vi "Autonomous Independent.vi"() -> ()   [LabVIEW 2015]
doc: "This VI is called when autonomous begins, and will automatically be terminated when autonomous ends. You can carry out timed or sensor driven robot movement independently without needing to return to the caller."
uses:
  <vilib>/Rock Robotics/WPI/SafetyOutput/WPI_SafetyOutputConfigMenu.ctl
  <vilib>/Rock Robotics/Network Tables/NT Read Number.vi
  <vilib>/Rock Robotics/WPI/Utilities/WPI_GetSetVariantRefNum.vi
  <vilib>/Rock Robotics/WPI/Solenoid/Deprecated/WPI_SolenoidGetBool.vi
  <vilib>/Rock Robotics/WPI/Solenoid/Deprecated/WPI_SolenoidSetBool.vi
panel:
  in  "Far":dbl=0.7
  in  "Close":dbl=0.7
  in  "Right Offset":dbl=1.0
  out "Defense Type":dbl=3.0
  in  "Auton_Modes":T1(array[cluster])=[{"Actions"=[{"Action"=enum."Drive", "Effort"=0.55, "Duration"=3.5}, {"Action"=enum."Nothing", "Effort"=0.0, "Duration"=0.0}]}, {"Actions"=[{"Action"=enum."Art Down", "Effort"=0.0, "Duration"=1.0}, {"Action"=enum."Drive", "Effort"=0.75, "Duration"=5.0}, {"Action"=enum."Art Up", "Effort"=0.0, "Duration"=1.0}]}, {"Actions"=[{"Action"=enum."Drive", "Effort"=1.0, "Duration"=3.0}, {"Action"=enum."Art Down", "Effort"=0.0, "Duration"=1.0}, {"Action"=enum."Drive", "Effort"=0.75, "Duration"=3.5}, {"Action"=enum."Art Up", "Effort"=0.0, "Duration"=1.0}]}, {"Actions"=[{"Action"=enum."Art Down", "Effort"=0.0, "Duration"=0.5}, {"Action"=enum."Drive", "Effort"=0.8, "Duration"=5.28}, {"Action"=enum."Art Up", "Effort"=0.0, "Duration"=1.0}, {"Action"=enum."Turn", "Effort"=-0.8, "Duration"=1.8}, {"Action"=enum."Nothing", "Effort"=0.0, "Duration"=0.1}, {"Action"=enum."Drive", "Effort"=0.8, "Duration"=1.75}, {"Action"=enum."Art Down", "Effort"=0.0, "Duration"=0.5}, {"Action"=enum."Vision Shot", "Effort"=0.0, "Duration"=4.0}]}, {"Actions"=[{"Action"=enum."Shift", "Effort"=0.0, "Duration"=0.0}, {"Action"=enum."Drive", "Effort"=1.0, "Duration"=0.1}, {"Action"=enum."Nothing", "Effort"=0.0, "Duration"=0.1}, {"Action"=enum."Drive", "Effort"=1.0, "Duration"=3.0}]}, {"Actions"=[{"Action"=enum."Shift", "Effort"=0.0, "Duration"=0.0}, {"Action"=enum."Drive", "Effort"=1.0, "Duration"=0.1}, {"Action"=enum."Nothing", "Effort"=0.0, "Duration"=0.1}, {"Action"=enum."Drive", "Effort"=1.0, "Duration"=3.0}]}, {"Actions"=[{"Action"=enum."Drive", "Effort"=0.55, "Duration"=4.0}, {"Action"=enum."Art Down", "Effort"=0.0, "Duration"=1.0}, {"Action"=enum."Drive", "Effort"=-0.5, "Duration"=0.6}, {"Action"=enum."Drive", "Effort"=0.75, "Duration"=1.0}, {"Action"=enum."Art Up", "Effort"=0.0, "Duration"=1.0}, {"Action"=enum."Drive", "Effort"=0.75, "Duration"=3.0}]}, {"Actions"=[{"Action"=enum."Art Down", "Effort"=0.0, "Duration"=0.5}, {"Action"=enum."Drive", "Effort"=0.55, "Duration"=4.25}, {"Action"=enum."Art Up", "Effort"=0.0, "Duration"=0.0}, {"Action"=enum."Nothing", "Effort"=0.0, "Duration"=0.3}, {"Action"=enum."Drive", "Effort"=0.9, "Duration"=2.0}]}, {"Actions"=[{"Action"=enum."Nothing", "Effort"=0.0, "Duration"=0.0}]}]
  # "0 Reach Defense\n1 Low Bar\n2 Rough Terrain\n3 Moat\n4 Rock Wall\n5 Ramparts\n6 Cheval\n7 Portcullis\n8 None"
  # "Reach"
  # "Low Bar"
  # "Rough Terrain"
  # "Moat"
  # "Low Bar \nVision"
  # "Rockwall"
  # "Left Side \nCheval w/\nTarget"
  # "Ramparts"
  # "Right Side \nCheval w/\ntarget"
  # "Cheval"
  # "Portcullis"
  # "None"
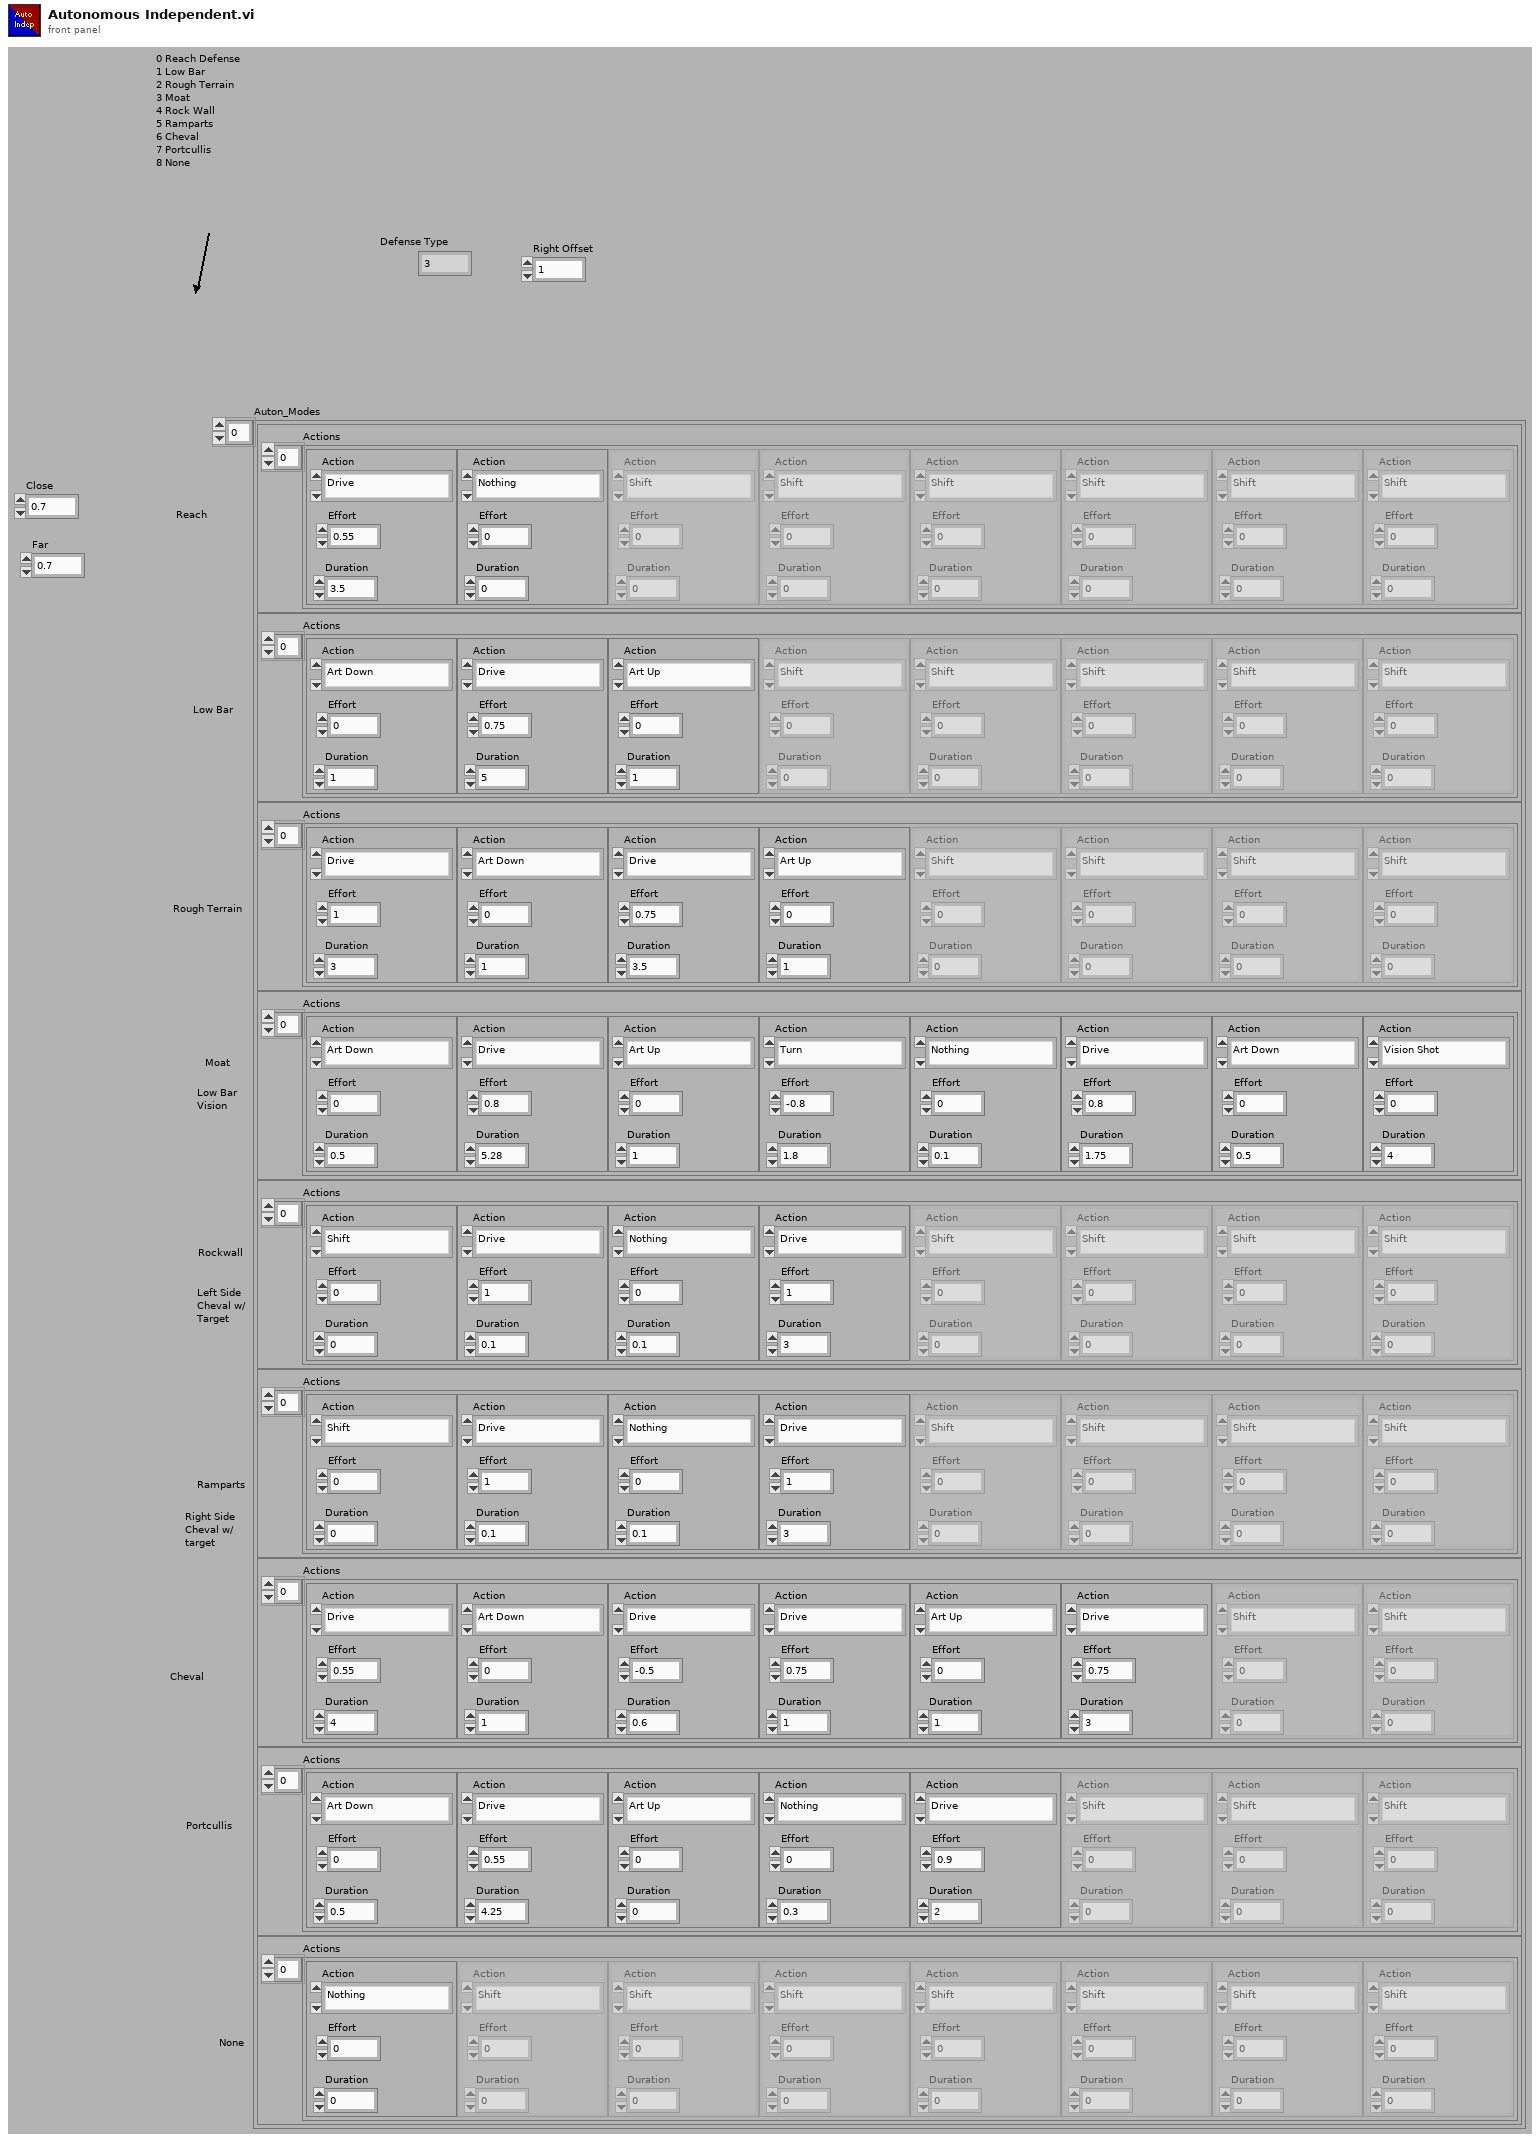
[diagram p1: front panel]
types:
  T1 = cluster{"Actions":cluster{"Action":enum16{"Shift", "Shoot", "Move Articulates", "Nothing", "Drive", "Turn", "Vision Shot", "Art Up", "Art Down", "Test"}, "Effort":dbl, "Duration":dbl}[]}[]
  T2 = cluster{"Actions":cluster{"Action":enum16{"Shift", "Shoot", "Move Articulates", "Nothing", "Drive", "Turn", "Vision Shot", "Art Up", "Art Down", "Test"}, "Effort":dbl, "Duration":dbl}[]}
  T3 = cluster{"Action":enum16{"Shift", "Shoot", "Move Articulates", "Nothing", "Drive", "Turn", "Vision Shot", "Art Up", "Art Down", "Test"}, "Effort":dbl, "Duration":dbl}[]
  T4 = typedef "WPI_SafetyOutputConfigMenu.ctl" = enum16{"Enable", "Disable"}
  T5 = enum16{"Shift", "Shoot", "Move Articulates", "Nothing", "Drive", "Turn", "Vision Shot", "Art Up", "Art Down", "Test"}
  T6 = typedef "WPI_RobotDriveDevRef.ctl" = cluster{"DevStatus":errorcluster, "Motors[]":T7[], "Square Inputs":bool, "Max Output":dbl}
  T7 = typedef "WPI_MotorControlDeviceRef.ctl" = cluster{"DeviceStatus":errorcluster, "Type":T8, "PWM":cluster{"PWM Channel":T9, "DeadBand":T10}, "CAN":cluster{"Device Number":u8, "Control Mode":T11, "Semaphore":T12, "Max Vout":dbl, "TalonSRX Control Mode":T13}, "Invert":bool}
  T8 = typedef "WPI_MotorControlType.ctl" = enum16{"PWM", "CAN", "CANTalonSRX"}
  T9 = typedef "FPGA_DIOPWMChannel.ctl" = enum8{"PWM 0", "PWM 1", "PWM 2", "PWM 3", "PWM 4", "PWM 5", "PWM 6", "PWM 7", "PWM 8", "PWM 9", "PWM MXP 0", "PWM MXP 1", "PWM MXP 2", "PWM MXP 3", "PWM MXP 4", "PWM MXP 5", "PWM MXP 6", "PWM MXP 7", "PWM MXP 8", "PWM MXP 9", "Invalid"}
  T10 = typedef "WPI_PWMDeadband.ctl" = cluster{"Name":string, "maxPositivePwm":i32, "minPositivePwm":i32, "centerPwm":i32, "maxNegativePwm":i32, "minNegativePwm":i32, "angularRange":u16}
  T11 = typedef "WPI_CANJaguar_ControlMode.ctl" = enum8{"Percent VBus", "Current", "Speed", "Position", "Voltage"}
  T12 = typedef "Semaphore RefNum" = refnum<k1>
  T13 = typedef "WPI_CANTalonSRX_APIControlMode.ctl" = enum8{"Percent VBus", "Speed", "Position", "Slave", "Unchanged / Invalid", "Voltage Compensation", "Current", "Motion Profile"}
  T14 = typedef "WPI_SolenoidDevRef.ctl" = cluster{"DevStatus":errorcluster, "Pneumatics Control Module":u8, "Forward Solenoid Channel":T15, "Reverse Solenoid Channel":T15}
  T15 = typedef "WPI_SolenoidChannel.ctl" = enum8{"Solenoid 0", "Solenoid 1", "Solenoid 2", "Solenoid 3", "Solenoid 4", "Solenoid 5", "Solenoid 6", "Solenoid 7", "Invalid"}
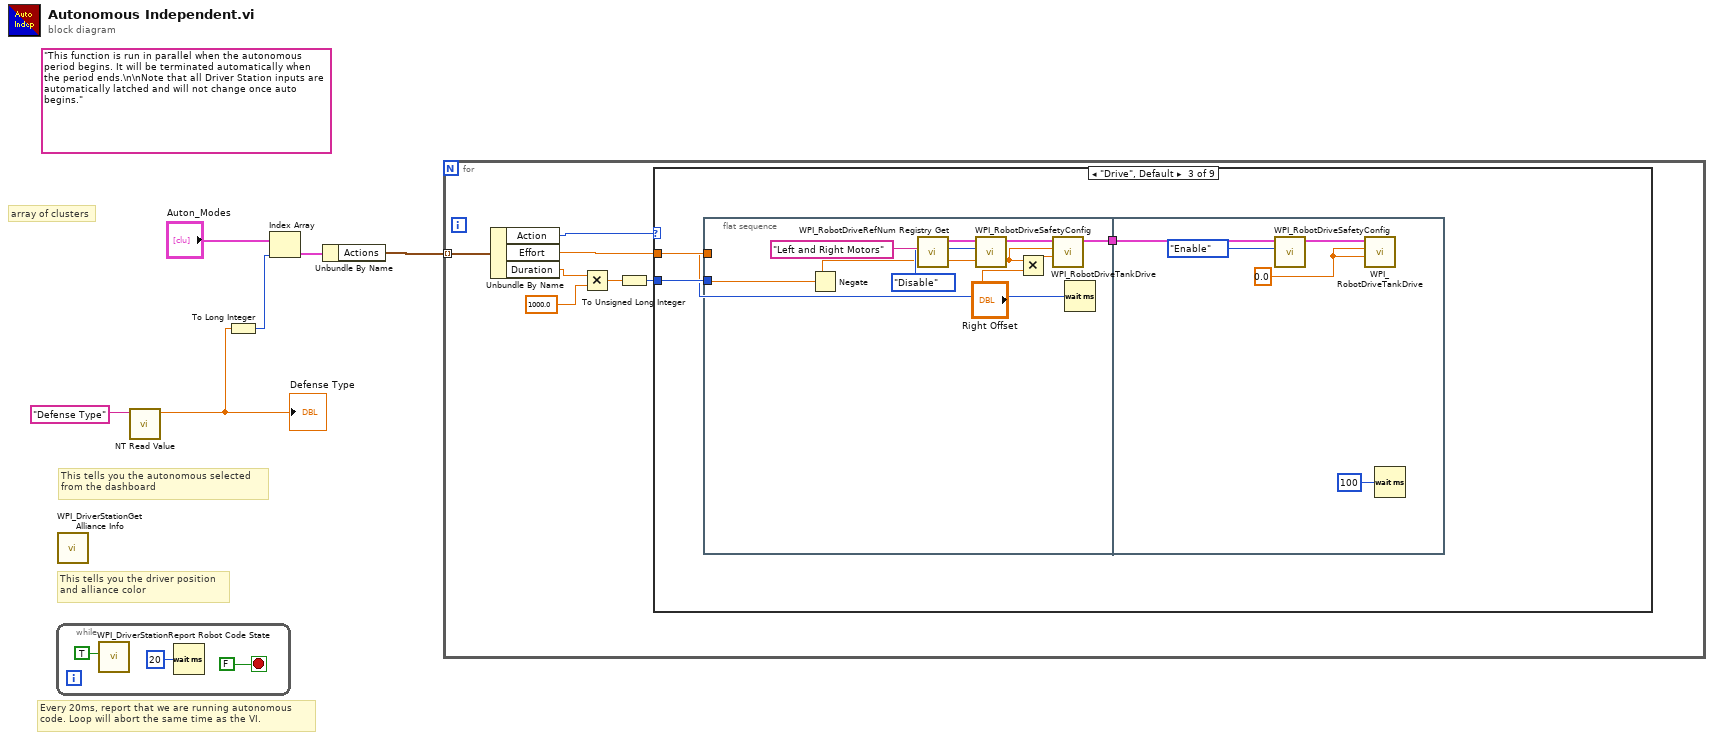
[diagram p0: block diagram]
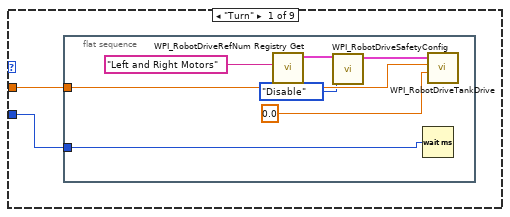
[diagram p2: hidden frame]
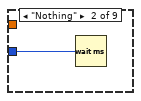
[diagram p3: hidden frame]
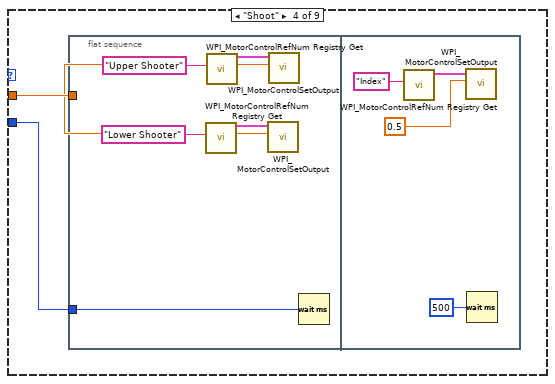
[diagram p4: hidden frame]
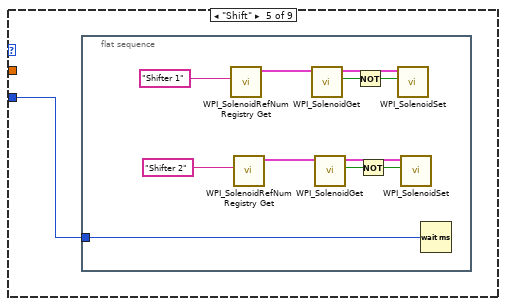
[diagram p5: hidden frame]
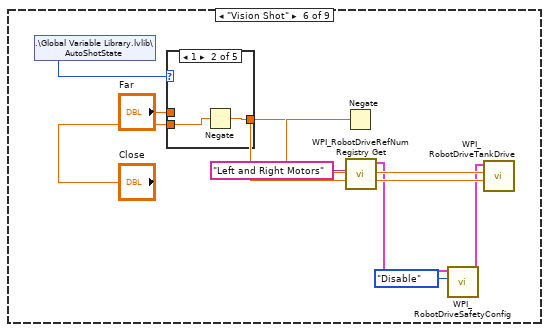
[diagram p6: hidden frame]
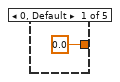
[diagram p7: hidden frame]
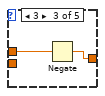
[diagram p8: hidden frame]
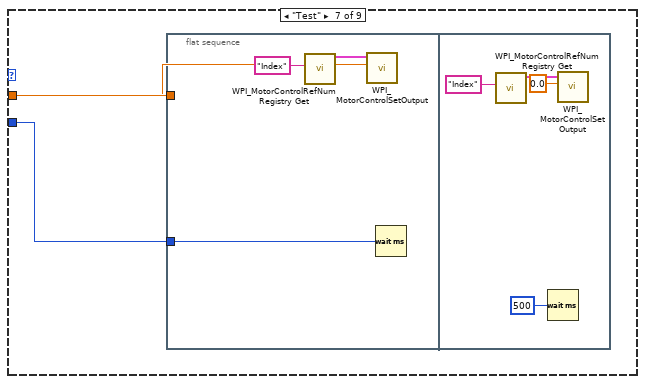
[diagram p11: hidden frame]
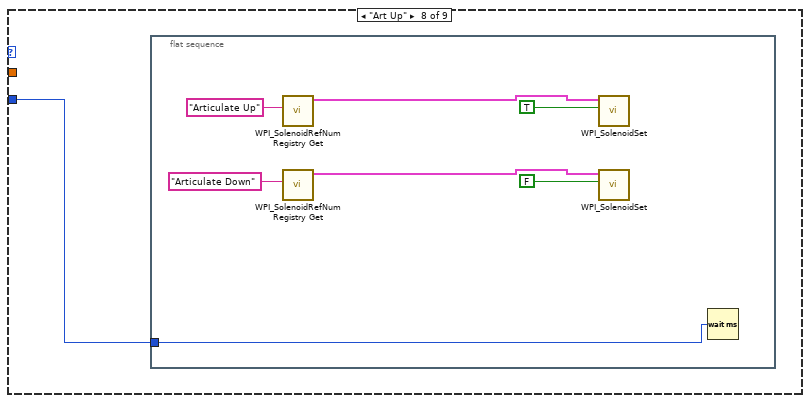
[diagram p12: hidden frame]
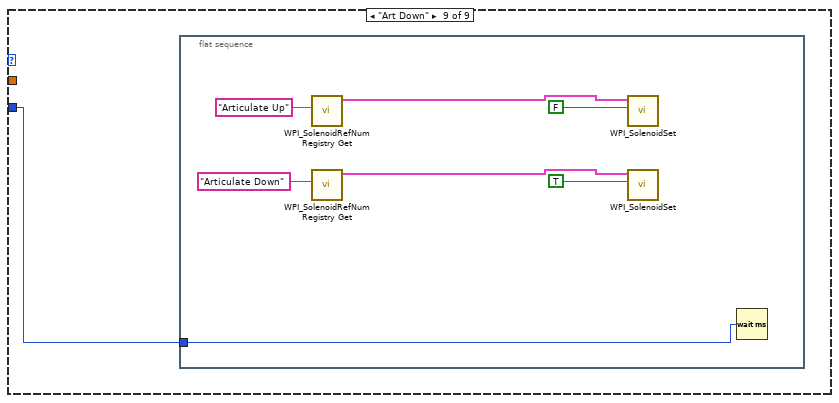
[diagram p13: hidden frame]
diagram:
  (unwired) "This function is run in parallel when the autonomous period begins. It will be terminated automatically when the period ends.\n\nNote that all Driver Station inputs are automatically latched and will not change once auto begins."
  # "This tells you the autonomous selected\nfrom the dashboard"
  # "array of clusters"
  # "Every 20ms, report that we are running autonomous\ncode. Loop will abort the same time as the VI."
  # "This tells you the driver position\nand alliance color"
  n1 = while {
    stop <- FALSE stop-if-true
    n2 = call <vilib>:"WPI_DriverStationReport Robot Code State.vi"("Autonomous"=TRUE) -> ()  [unwired: 10 in, 1 out]
    n3 = Wait (ms)(milliseconds to wait=u32 20) -> ()  [unwired: 1 out]
  }
  n4 = call <vilib>:"WPI_DriverStationGet Alliance Info.vi"() -> ()  [unwired: 12 out]
  n5 = call-poly <vilib>:"NT Read Value.vi"("Name"="Defense Type") -> ("Numeric"=w1:dbl)  [unwired: 9 in, 1 out]
  "Defense Type" <- w1
  n6 = To Long Integer(number=w1) -> (32bit integer=w3:i32)
  n7 = Index Array(array="Auton_Modes", index=w3) -> (element=w5:T2)
  n8 = Unbundle By Name(w5) -> ("Actions"=w6:T3)
  n9 = for {
    tunnel: w6 -> [w16] mode=indexing
    n10 = Unbundle By Name(w16) -> ("Action"=w15:T5, "Effort"=w14:dbl, "Duration"=w13:dbl)
    n11 = Multiply(x=w13, y=1000.0) -> (x*y=w10:dbl)
    n12 = To Unsigned Long Integer(number=w10) -> (unsigned 32bit integer=w11:u32)
    n13 = case shown="\"Drive\", Default" w15 {
      tunnel: w14 -> [w18 _ w29 w45 _ _ w86 _ _]
      tunnel: w11 -> [w17 w26 w28 w46 w57 _ w85 w95 w103]
      frame "Turn" {
        n14 = flat-sequence {
          tunnel: w18 -> [w23]
          tunnel: w17 -> [w24]
          frame #0 {
            n15 = call <vilib>:"WPI_RobotDriveRefNum Registry Get.vi"("refnum name"="Left and Right Motors") -> ("RobotDriveDevRef"=w21:T6)  [unwired: 9 in, 1 out]
            n16 = call <vilib>:"WPI_RobotDriveSafetyConfig.vi"("mode"=WPI_SafetyOutputConfigMenu."Disable", "RobotDriveDevRef"=w21) -> ("RobotDriveDevRef"=w20:T6)  [unwired: 8 in, 1 out]
            n17 = Wait (ms)(milliseconds to wait=w24) -> ()  [unwired: 1 out]
            n18 = call <vilib>:"WPI_RobotDriveTankDrive.vi"("Right axis value"=0.0, "Left axis value"=w23, "RobotDriveDevRef"=w20) -> ()  [unwired: 6 in, 3 out]
          }
        }
      }
      frame "Nothing" {
        n19 = Wait (ms)(milliseconds to wait=w26) -> ()  [unwired: 1 out]
      }
      frame "Drive", Default {
        n20 = flat-sequence {
          tunnel: w29 -> [w37]
          tunnel: w28 -> [w36]
          tunnel: [w35] -> w27
          tunnel: w27 -> [w42]
          frame #0 {
            n21 = Negate(x=w37) -> (-x=w31:dbl)
            n22 = call <vilib>:"WPI_RobotDriveRefNum Registry Get.vi"("refnum name"="Left and Right Motors") -> ("RobotDriveDevRef"=w38:T6)  [unwired: 9 in, 1 out]
            n23 = call <vilib>:"WPI_RobotDriveSafetyConfig.vi"("mode"=WPI_SafetyOutputConfigMenu."Disable", "RobotDriveDevRef"=w38) -> ("RobotDriveDevRef"=w34:T6)  [unwired: 8 in, 1 out]
            n24 = Multiply(x=w31, y="Right Offset") -> (x*y=w32:dbl)
            n25 = call <vilib>:"WPI_RobotDriveTankDrive.vi"("Right axis value"=w32, "Left axis value"=w31, "RobotDriveDevRef"=w34) -> ("RobotDriveDevRef"=w35:T6)  [unwired: 6 in, 2 out]
            n26 = Wait (ms)(milliseconds to wait=w36) -> ()  [unwired: 1 out]
          }
          frame #1 {
            w44 = 0.0
            n27 = call <vilib>:"WPI_RobotDriveSafetyConfig.vi"("mode"=WPI_SafetyOutputConfigMenu."Enable", "RobotDriveDevRef"=w42) -> ("RobotDriveDevRef"=w41:T6)  [unwired: 8 in, 1 out]
            n28 = call <vilib>:"WPI_RobotDriveTankDrive.vi"("Right axis value"=w44, "Left axis value"=w44, "RobotDriveDevRef"=w41) -> ()  [unwired: 6 in, 3 out]
            n29 = Wait (ms)(milliseconds to wait=u32 100) -> ()  [unwired: 1 out]
          }
        }
      }
      frame "Shoot" {
        n30 = flat-sequence {
          tunnel: w46 -> [w47]
          tunnel: w45 -> [w48]
          frame #0 {
            n31 = call <vilib>:"WPI_MotorControlRefNum Registry Get.vi"("refnum name"="Lower Shooter") -> ("MotorControlDevRef"=w49:T7)  [unwired: 9 in, 1 out]
            n32 = call <vilib>:"WPI_MotorControlRefNum Registry Get.vi"("refnum name"="Upper Shooter") -> ("MotorControlDevRef"=w52:T7)  [unwired: 9 in, 1 out]
            n33 = call <vilib>:"WPI_MotorControlSetOutput.vi"("Output"=w48, "MotorControlDevRef"=w49) -> ()  [unwired: 7 in, 3 out]
            n34 = call <vilib>:"WPI_MotorControlSetOutput.vi"("Output"=w48, "MotorControlDevRef"=w52) -> ()  [unwired: 7 in, 3 out]
            n35 = Wait (ms)(milliseconds to wait=w47) -> ()  [unwired: 1 out]
          }
          frame #1 {
            n36 = call <vilib>:"WPI_MotorControlRefNum Registry Get.vi"("refnum name"="Index") -> ("MotorControlDevRef"=w55:T7)  [unwired: 9 in, 1 out]
            n37 = call <vilib>:"WPI_MotorControlSetOutput.vi"("Output"=0.5, "MotorControlDevRef"=w55) -> ()  [unwired: 7 in, 3 out]
            n38 = Wait (ms)(milliseconds to wait=u32 500) -> ()  [unwired: 1 out]
          }
        }
      }
      frame "Shift" {
        n39 = flat-sequence {
          tunnel: w57 -> [w58]
          frame #0 {
            n40 = call <vilib>:"WPI_SolenoidRefNum Registry Get.vi"("refnum name"="Shifter 1") -> ("SolenoidDevRef"=w68:T14)  [unwired: 9 in, 1 out]
            n41 = call <vilib>:"WPI_SolenoidRefNum Registry Get.vi"("refnum name"="Shifter 2") -> ("SolenoidDevRef"=w59:T14)  [unwired: 9 in, 1 out]
            n42 = call-poly <vilib>:"WPI_SolenoidGet.vi"("SolenoidDevRef"=w68) -> ("Value"=w66:bool, "SolenoidDevRef"=w67:T14)  [unwired: 8 in, 1 out]
            n43 = call-poly <vilib>:"WPI_SolenoidGet.vi"("SolenoidDevRef"=w59) -> ("Value"=w61:bool, "SolenoidDevRef"=w60:T14)  [unwired: 8 in, 1 out]
            n44 = Not(x=w66) -> (.not. x?=w64:bool)
            n45 = Not(x=w61) -> (.not. x?=w63:bool)
            n46 = call-poly <vilib>:"WPI_SolenoidSet.vi"("Value"=w64, "SolenoidDevRef"=w67) -> ()  [unwired: 8 in, 2 out]
            n47 = call-poly <vilib>:"WPI_SolenoidSet.vi"("Value"=w63, "SolenoidDevRef"=w60) -> ()  [unwired: 8 in, 2 out]
            n48 = Wait (ms)(milliseconds to wait=w58) -> ()  [unwired: 1 out]
          }
        }
      }
      frame "Vision Shot" {
        n49 = shared-variable ".\\Global Variable Library.lvlib\\AutoShotState"() -> (w75:u32)  [unwired: 1 in, 1 out]
        n50 = case shown="1" w75 {
          tunnel: [0.0 w80 w82 w83 w84] -> w72
          tunnel: "Far" -> [_ _ w81 _ w84]
          tunnel: "Close" -> [_ w79 _ w83 _]
          frame 0, Default {
          }
          frame 1 {
            n51 = Negate(x=w79) -> (-x=w80:dbl)
          }
          frame 3 {
            n52 = Negate(x=w81) -> (-x=w82:dbl)
          }
          frame 4 {
          }
          frame 6 {
          }
        }
        n53 = Negate(x=w72) -> (-x=w77:dbl)
        n54 = call <vilib>:"WPI_RobotDriveRefNum Registry Get.vi"("refnum name"="Left and Right Motors") -> ("RobotDriveDevRef"=w71:T6)  [unwired: 9 in, 1 out]
        n55 = call <vilib>:"WPI_RobotDriveSafetyConfig.vi"("mode"=WPI_SafetyOutputConfigMenu."Disable", "RobotDriveDevRef"=w71) -> ("RobotDriveDevRef"=w70:T6)  [unwired: 8 in, 1 out]
        n56 = call <vilib>:"WPI_RobotDriveTankDrive.vi"("Right axis value"=w72, "Left axis value"=w77, "RobotDriveDevRef"=w70) -> ()  [unwired: 6 in, 3 out]
      }
      frame "Test" {
        n57 = flat-sequence {
          tunnel: w86 -> [w88]
          tunnel: w85 -> [w87]
          frame #0 {
            n58 = call <vilib>:"WPI_MotorControlRefNum Registry Get.vi"("refnum name"="Index") -> ("MotorControlDevRef"=w90:T7)  [unwired: 9 in, 1 out]
            n59 = call <vilib>:"WPI_MotorControlSetOutput.vi"("Output"=w88, "MotorControlDevRef"=w90) -> ()  [unwired: 7 in, 3 out]
            n60 = Wait (ms)(milliseconds to wait=w87) -> ()  [unwired: 1 out]
          }
          frame #1 {
            n61 = call <vilib>:"WPI_MotorControlRefNum Registry Get.vi"("refnum name"="Index") -> ("MotorControlDevRef"=w93:T7)  [unwired: 9 in, 1 out]
            n62 = Wait (ms)(milliseconds to wait=u32 500) -> ()  [unwired: 1 out]
            n63 = call <vilib>:"WPI_MotorControlSetOutput.vi"("Output"=0.0, "MotorControlDevRef"=w93) -> ()  [unwired: 7 in, 3 out]
          }
        }
      }
      frame "Art Up" {
        n64 = flat-sequence {
          tunnel: w95 -> [w96]
          frame #0 {
            n65 = call <vilib>:"WPI_SolenoidRefNum Registry Get.vi"("refnum name"="Articulate Up") -> ("SolenoidDevRef"=w100:T14)  [unwired: 9 in, 1 out]
            n66 = call <vilib>:"WPI_SolenoidRefNum Registry Get.vi"("refnum name"="Articulate Down") -> ("SolenoidDevRef"=w97:T14)  [unwired: 9 in, 1 out]
            n67 = call-poly <vilib>:"WPI_SolenoidSet.vi"("Value"=TRUE, "SolenoidDevRef"=w100) -> ()  [unwired: 8 in, 2 out]
            n68 = call-poly <vilib>:"WPI_SolenoidSet.vi"("Value"=FALSE, "SolenoidDevRef"=w97) -> ()  [unwired: 8 in, 2 out]
            n69 = Wait (ms)(milliseconds to wait=w96) -> ()  [unwired: 1 out]
          }
        }
      }
      frame "Art Down" {
        n70 = flat-sequence {
          tunnel: w103 -> [w104]
          frame #0 {
            n71 = call <vilib>:"WPI_SolenoidRefNum Registry Get.vi"("refnum name"="Articulate Up") -> ("SolenoidDevRef"=w108:T14)  [unwired: 9 in, 1 out]
            n72 = call <vilib>:"WPI_SolenoidRefNum Registry Get.vi"("refnum name"="Articulate Down") -> ("SolenoidDevRef"=w105:T14)  [unwired: 9 in, 1 out]
            n73 = call-poly <vilib>:"WPI_SolenoidSet.vi"("Value"=FALSE, "SolenoidDevRef"=w108) -> ()  [unwired: 8 in, 2 out]
            n74 = call-poly <vilib>:"WPI_SolenoidSet.vi"("Value"=TRUE, "SolenoidDevRef"=w105) -> ()  [unwired: 8 in, 2 out]
            n75 = Wait (ms)(milliseconds to wait=w104) -> ()  [unwired: 1 out]
          }
        }
      }
    }
  }
